vi "SIM_PeriodicTasks.vi"(8 "error in":errorcluster) -> ()   [LabVIEW 2025]
doc: "This VI runs in parallel to other tasks. It can contain as many user-defined periodic loops as you need. These can carry out PID or other sorts of timed response."
uses:
  <vilib>/Rock Robotics/WPI/ThirdParty/PhotonVisionLib/PhotonVisionLib.lvlib
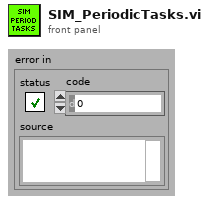
[diagram p1: front panel]
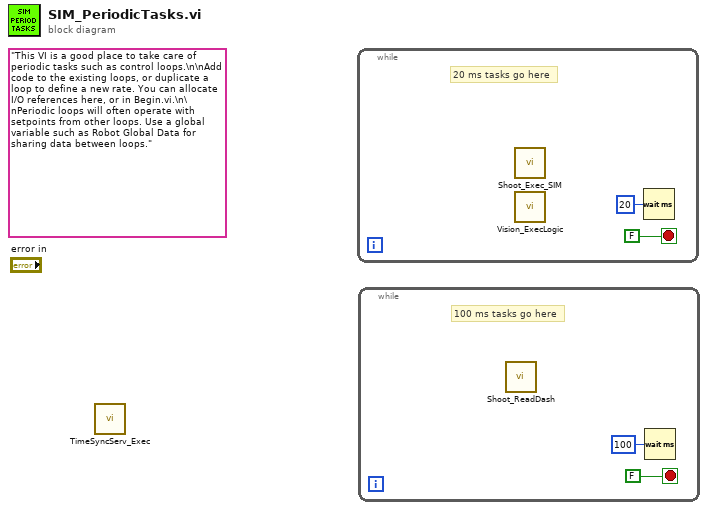
[diagram p0: block diagram]
diagram:
  (unwired) "This VI is a good place to take care of periodic tasks such as control loops.\n\nAdd code to the existing loops, or duplicate a loop to define a new rate. You can allocate I/O references here, or in Begin.vi.\n\nPeriodic loops will often operate with setpoints from other loops. Use a global variable such as Robot Global Data for sharing data between loops."
  n1 = call <vilib>:"TimeSyncServ_Exec.vi"() -> ()  [unwired: 12 in]
  n2 = while {
    stop <- FALSE stop-if-true
    # "20 ms tasks go here"
    n3 = call "Shoot_Exec_SIM.vi"() -> ()  [unwired: 12 in]
    n4 = call "Vision_ExecLogic.vi"() -> ()  [unwired: 12 in]
    n5 = Wait (ms)(milliseconds to wait=u32 20) -> ()  [unwired: 1 out]
  }
  n6 = while {
    stop <- FALSE stop-if-true
    # "100 ms tasks go here"
    n7 = call "Shoot_ReadDash.vi"() -> ()  [unwired: 12 in]
    n8 = Wait (ms)(milliseconds to wait=u32 100) -> ()  [unwired: 1 out]
  }
